vi "Write Frequency.vi"(8 "error in (no error)":errorcluster, 10 "Frequency":dbl, 11 "Composite Waveform in":refnum<class "Composite Waveform.lvclass">) -> (0 "error out":errorcluster, 3 "Composite Waveform out":refnum<class "Composite Waveform.lvclass">)   [LabVIEW 2020, in "Composite Waveform.lvclass"]
uses:
  Composite Waveform.lvclass
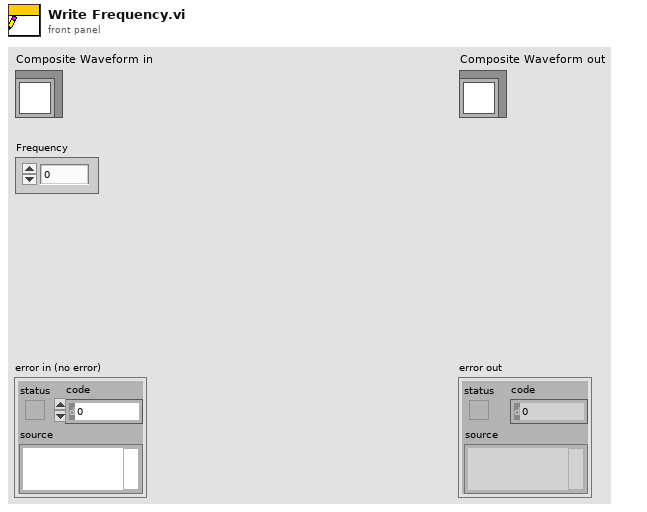
[diagram p1: front panel]
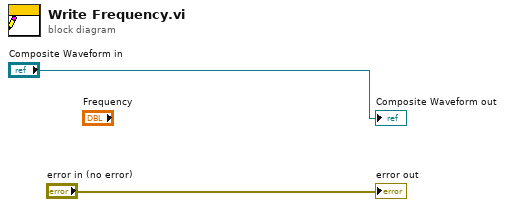
[diagram p0: block diagram]
diagram:
  "error out" <- "error in (no error)"
  "Composite Waveform out" <- "Composite Waveform in"
